vi "TagBus_Cluster to TagBus Index (DVR).vi"(7 "Clust Refnum":refnum<vi>, 10 "Tag Name Prepend":string, 11 "TagBus DVR":refnum<data-value>) -> (2 "Index Array":i32[](array[numeric]), 3 "TagBus DVR out":refnum<data-value>)   [LabVIEW 2015, in "TagBus.lvclass"]
uses:
  TagBus.lvclass
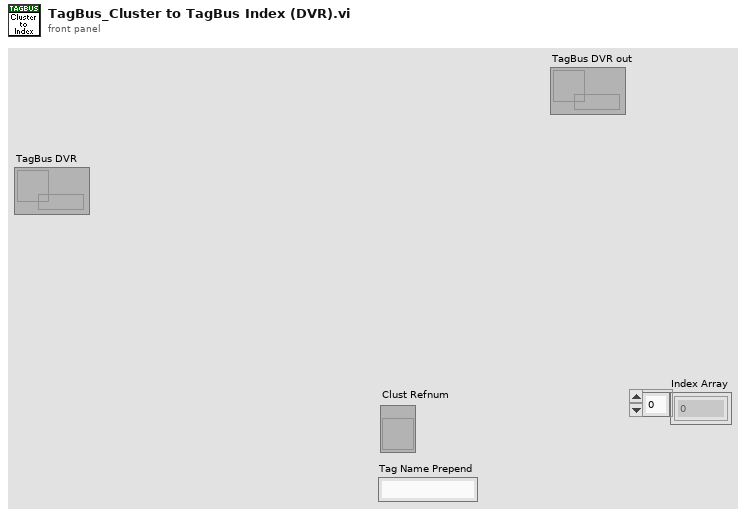
[diagram p1: front panel]
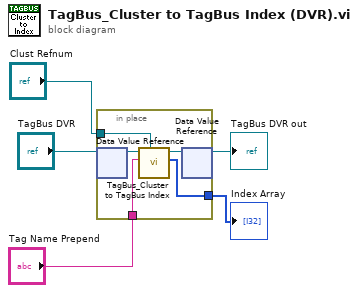
[diagram p0: block diagram]
diagram:
  n1 = in-place {
    in-place-border: "Clust Refnum" -> [w7]
    in-place-border: [w8] -> w5
    in-place-border: "Tag Name Prepend" -> [w6]
    n2 = in-place-dvr #1("TagBus DVR") -> (w10:refnum<class "TagBus.lvclass">)  [unwired: 1 out]
    n3 = call "TagBus_Cluster to TagBus Index.vi"("Clust Refnum"=w7, "Process Name Modifier"=w6, "TagBus"=w10) -> ("Index Array"=w8:i32[], "TagBus out"=w9:refnum<class "TagBus.lvclass">)  [unwired: 7 in]
    n4 = in-place-dvr #1(w9) -> (→"TagBus DVR out":refnum<data-value>)  [unwired: 1 out]
  }
  "Index Array" <- w5
